vi "ADC to Volts.vi"(2 "maxValue":u16, 3 "ADC values":u16[](array[numeric])) -> (1 "values in Volt":dbl[](array[numeric]))   [LabVIEW 2010]
doc: "Converts the raw ADC readings to values in Volt.\n\n<b>maxValue</b> is the output of pl1000MaxValue.vi"
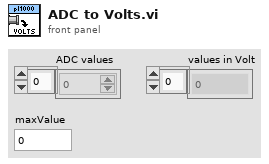
[diagram p1: front panel]
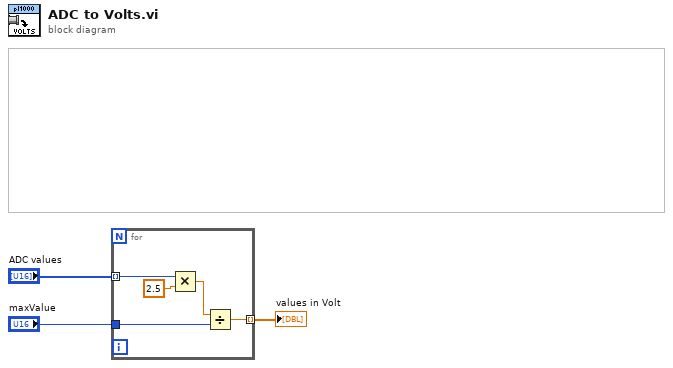
[diagram p0: block diagram]
diagram:
  n1 = for {
    tunnel: "ADC values" -> [w8] mode=indexing
    tunnel: "maxValue" -> [w5]
    tunnel: [w4] -> w1 mode=indexing
    n2 = Multiply(x=w8, y=2.5) -> (x*y=w6:dbl)
    n3 = Divide(x=w6, y=w5) -> (x/y=w4:dbl)
  }
  "values in Volt" <- w1
